vi "Save Macro Steps.vi"(8 "error in (no error)":errorcluster, 10 "Macro Steps":T1[](array[typedef]), 11 "refnum":T3) -> (0 "error out":errorcluster, 3 "refnum out":T3)   [LabVIEW 2020, in "MacroAssert.lvlib"]
doc: "Saves the list of steps to the macro config file defined by <B>refnum</B>."
uses:
  MacroAssert.lvlib
  <vilib>/Utility/config.llb/Config Data RefNum.ctl
  CTLs/Step V3.ctl
  CTLs/Step Type V3.ctl
  <vilib>/Utility/config.llb/Write Key (I32).vi
  <vilib>/Utility/config.llb/Write Key (String).vi
  <vilib>/Utility/config.llb/Write Key (Boolean).vi
  <vilib>/Utility/config.llb/Write Key (U32).vi
  <vilib>/Utility/config.llb/NI_LVConfig.lvlib
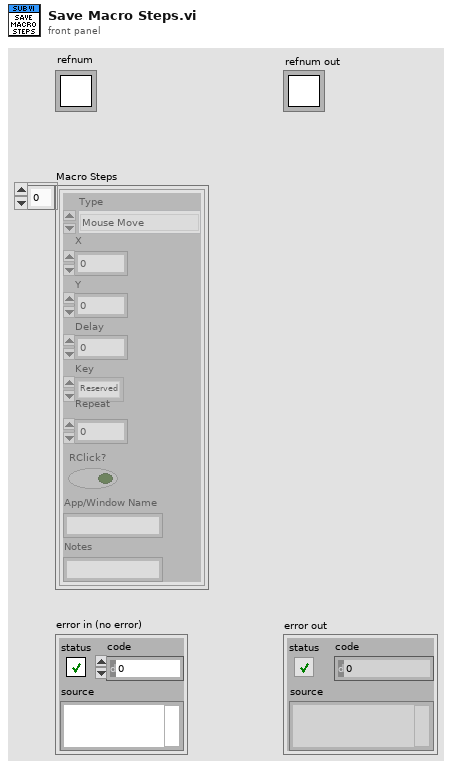
[diagram p1: front panel]
types:
  T1 = typedef "MacroAssert.lvlib/Step V3.ctl" = cluster{"Type":T2, "X":i32, "Y":i32, "Delay":i32, "Key":u8, "Repeat":i32, "RClick?":bool, "App/Window Name":string, "Notes":string}
  T2 = typedef "MacroAssert.lvlib/Step Type V3.ctl" = enum16{"Mouse Move", "Mouse Click", "Key Press", "Wait", "Mouse Down", "Mouse Up", "Key Down", "Key Up", "Run Application", "Maximize Window", "Restore Window", "Minimize Window", "Close Window", "Bring Window to Front", "Send Window to Back"}
  T3 = typedef "NI_LVConfig.lvlib/Config Data RefNum.ctl" = refnum<k1>
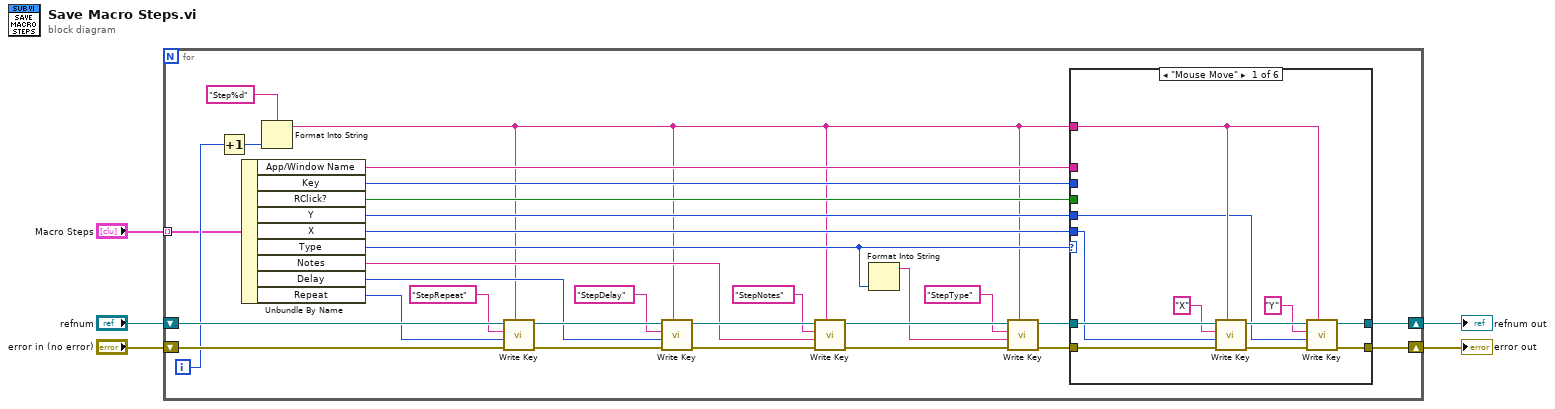
[diagram p0: block diagram]
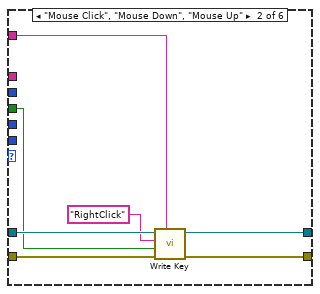
[diagram p2: hidden frame]
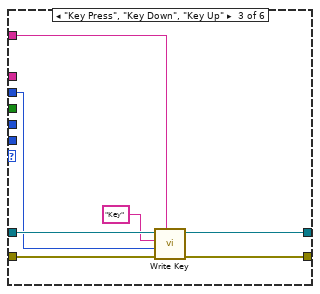
[diagram p3: hidden frame]
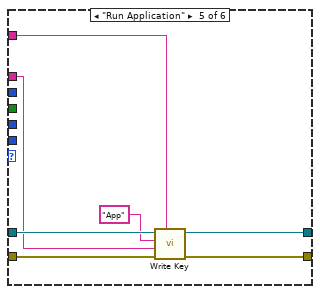
[diagram p5: hidden frame]
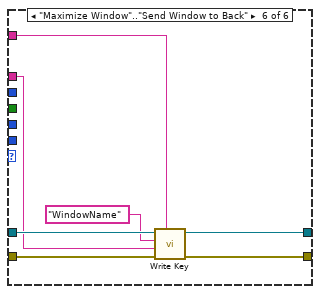
[diagram p6: hidden frame]
diagram:
  n1 = for {
    shift-right: [w29] -> w2
    shift-left: "error in (no error)" -> [w34]
    shift-right: [w28] -> w1
    shift-left: "refnum" -> [w31]
    tunnel: "Macro Steps" -> [w16] mode=indexing
    i -> [w26]
    n2 = Increment(x=w26) -> (x+1=w25:i32)
    n3 = Unbundle By Name(w16) -> ("App/Window Name"=w11:string, "Key"=w12:u8, "RClick?"=w13:bool, "Y"=w14:i32, "X"=w15:i32, "Type"=w21:T2, "Notes"=w7:string, "Delay"=w17:i32, "Repeat"=w18:i32)
    n4 = Format Into String(format string="Step%d", w25) -> (resulting string=w6:string)  [unwired: 2 in, 1 out]
    n5 = call-poly <vilib>:"Write Key.vi"("section"=w6, "error in (no error)"=w34, "value"=w18, "key"="StepRepeat", "refnum"=w31) -> ("error out"=w35:errorcluster, "refnum out"=w32:T3)  [unwired: 4 in, 1 out]
    n6 = call-poly <vilib>:"Write Key.vi"("section"=w6, "error in (no error)"=w35, "value"=w17, "key"="StepDelay", "refnum"=w32) -> ("error out"=w33:errorcluster, "refnum out"=w9:T3)  [unwired: 4 in, 1 out]
    n7 = call-poly <vilib>:"Write Key.vi"("section"=w6, "error in (no error)"=w33, "value"=w7, "key"="StepNotes", "refnum"=w9) -> ("error out"=w10:errorcluster, "refnum out"=w36:T3)  [unwired: 4 in, 1 out]
    n8 = Format Into String(w21) -> (resulting string=w23:string)  [unwired: 3 in, 1 out]
    n9 = call-poly <vilib>:"Write Key.vi"("section"=w6, "error in (no error)"=w10, "value"=w23, "key"="StepType", "refnum"=w36) -> ("error out"=w20:errorcluster, "refnum out"=w19:T3)  [unwired: 4 in, 1 out]
    n10 = case shown="\"Mouse Move\"" w21 {
      tunnel: w20 -> [w46 w54 w61 w62 w70 w77]
      tunnel: w19 -> [w45 w53 w60 w63 w69 w76]
      tunnel: w6 -> [w41 w51 w58 _ w67 w74]
      tunnel: [w40 w49 w56 w62 w65 w72] -> w29
      tunnel: [w39 w50 w57 w63 w66 w73] -> w28
      tunnel: w15 -> [w38 _ _ _ _ _]
      tunnel: w14 -> [w37 _ _ _ _ _]
      tunnel: w13 -> [_ w48 _ _ _ _]
      tunnel: w12 -> [_ _ w55 _ _ _]
      tunnel: w11 -> [_ _ _ _ w64 w71]
      frame "Mouse Move" {
        n11 = call-poly <vilib>:"Write Key.vi"("section"=w41, "error in (no error)"=w46, "value"=w38, "key"="X", "refnum"=w45) -> ("error out"=w42:errorcluster, "refnum out"=w47:T3)  [unwired: 4 in, 1 out]
        n12 = call-poly <vilib>:"Write Key.vi"("section"=w41, "error in (no error)"=w42, "value"=w37, "key"="Y", "refnum"=w47) -> ("error out"=w40:errorcluster, "refnum out"=w39:T3)  [unwired: 4 in, 1 out]
      }
      frame "Mouse Click", "Mouse Down", "Mouse Up" {
        n13 = call-poly <vilib>:"Write Key.vi"("section"=w51, "error in (no error)"=w54, "value"=w48, "key"="RightClick", "refnum"=w53) -> ("error out"=w49:errorcluster, "refnum out"=w50:T3)  [unwired: 4 in, 1 out]
      }
      frame "Key Press", "Key Down", "Key Up" {
        n14 = call-poly <vilib>:"Write Key.vi"("section"=w58, "error in (no error)"=w61, "value"=w55, "key"="Key", "refnum"=w60) -> ("error out"=w56:errorcluster, "refnum out"=w57:T3)  [unwired: 4 in, 1 out]
      }
      frame "Wait" {
      }
      frame "Run Application" {
        n15 = call-poly <vilib>:"Write Key.vi"("section"=w67, "error in (no error)"=w70, "value"=w64, "key"="App", "refnum"=w69) -> ("error out"=w65:errorcluster, "refnum out"=w66:T3)  [unwired: 4 in, 1 out]
      }
      frame "Maximize Window".."Send Window to Back" {
        n16 = call-poly <vilib>:"Write Key.vi"("section"=w74, "error in (no error)"=w77, "value"=w71, "key"="WindowName", "refnum"=w76) -> ("error out"=w72:errorcluster, "refnum out"=w73:T3)  [unwired: 4 in, 1 out]
      }
    }
  }
  "error out" <- w2
  "refnum out" <- w1
